vi "Explorer_SplitRows.vi"(11 "Array in":dbl[][](array[numeric])) -> (3 "XY Plot":cluster{dbl[], dbl[]}[](graph))   [LabVIEW 2021]
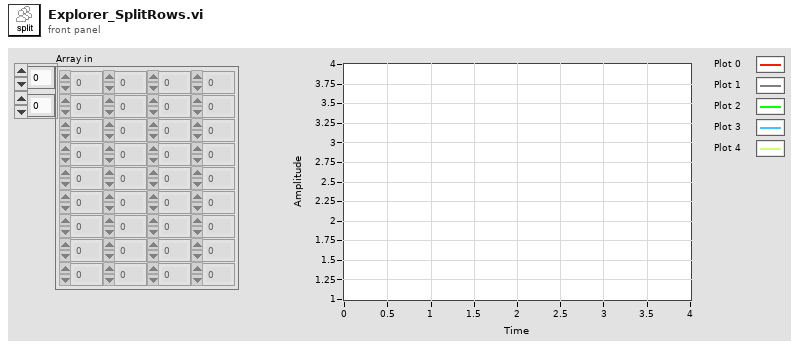
[diagram p1: front panel]
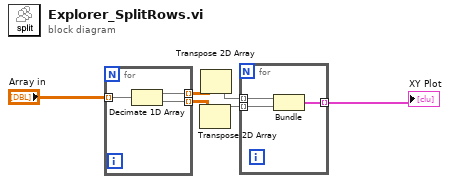
[diagram p0: block diagram]
diagram:
  n1 = for {
    tunnel: "Array in" -> [w9] mode=indexing
    tunnel: [w8] -> w4 mode=indexing
    tunnel: [w7] -> w5 mode=indexing
    n2 = Decimate 1D Array(w9) -> (w8:dbl[], w7:dbl[])
  }
  n3 = Transpose 2D Array(2D array=w5) -> (transposed array=w2:dbl[][])
  n4 = Transpose 2D Array(2D array=w4) -> (transposed array=w3:dbl[][])
  n5 = for {
    tunnel: w3 -> [w12] mode=indexing
    tunnel: w2 -> [w11] mode=indexing
    tunnel: [w10] -> w1 mode=indexing
    n6 = Bundle(w12, w11) -> (w10:cluster{dbl[], dbl[]})  [unwired: 1 in]
  }
  "XY Plot" <- w1
